vi "Teleop.vi"(10 "Match Info":T1={"Autonomous Elapsed Seconds"=0.0, "TeleOp Elapsed Seconds"=0.0, "Disabled Elapsed Seconds"=0.0, "Visited Autonomous"=FALSE, "Visited TeleOp"=FALSE, "Visited Disabled"=FALSE, "Autonomous Settings"={"Autonomous Style"=enum."Independent", "VI Refnum"=refnum}}, 11 "Call Context":T2) -> ()   [LabVIEW 2013]
doc: "This VI is called for each TeleOp packet received from the DS where the robot is not disabled. It is often used to read from the joysticks and update I/O or to update setpoints for timed control loops. It should complete and return within 20 milliseconds or it may miss DS packets."
uses:
  <vilib>/Rock Robotics/WPI/DriverStation/WPI_DriverStationDerivedRobotMode.ctl
  <vilib>/Rock Robotics/WPI/DriverStation/WPI_DriverStationMatch Info.ctl
  <vilib>/Rock Robotics/WPI/Relay/WPI_RelayValue.ctl
  Robot Global Data.vi
  <vilib>/Rock Robotics/WPI/Joystick/WPI_JoystickGetSetRefNum.vi
  <vilib>/Rock Robotics/WPI/Compressor/WPI_CompressorGetSetRefNum.vi
panel:
  in  "Release to Retract":u32=750
  in  "Time Between Open and Shoot":u32=250
  in  "GO BUTTON?":bool
  out "Numeric 1":dbl(slide) scale=0.0..100.0
  out "Boolean 2":bool
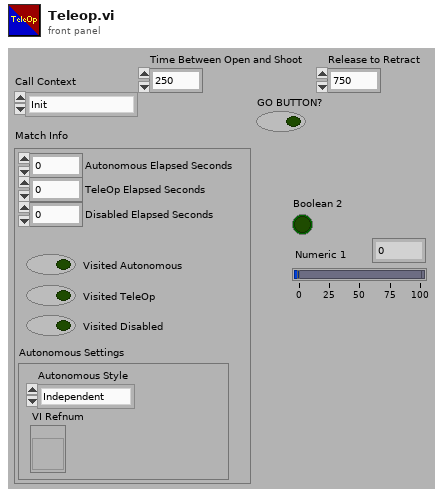
[diagram p1: front panel]
types:
  T1 = typedef "WPI_DriverStationMatch Info.ctl" = cluster{"Autonomous Elapsed Seconds":dbl, "TeleOp Elapsed Seconds":dbl, "Disabled Elapsed Seconds":dbl, "Visited Autonomous":bool, "Visited TeleOp":bool, "Visited Disabled":bool, "Autonomous Settings":cluster{"Autonomous Style":enum16{"Iterative", "Independent"}, "VI Refnum":refnum<vi>}}
  T2 = typedef "WPI_DriverStationDerivedRobotMode.ctl" = enum16{"Init", "Execute", "Stop"}
  T3 = typedef "WPI_RelayValue.ctl" = enum16{"Off", "On", "Forward", "Reverse"}
  T4 = typedef "WPI_JoystickDevRef.ctl" = cluster{"Device":T5}
  T5 = typedef "WPI_JoystickDeviceEnum.ctl" = enum16{"USB 1", "USB 2", "USB 3", "USB 4", "Kinect 1", "Kinect 2"}
  T6 = typedef "WPI_JoystickButtonState.ctl" = cluster{"Button 1":bool, "Button 2":bool, "Button 3":bool, "Button 4":bool, "Button 5":bool, "Button 6":bool, "Button 7":bool, "Button 8":bool, "Button 9":bool, "Button 10":bool, "Button 11":bool, "Button 12":bool}
  T7 = cluster{"axis 1 (x)":dbl, "axis 2 (y)":dbl, "axis 3 (throttle)":dbl, "axis 4":dbl, "axis 5":dbl, "axis 6":dbl}
  T8 = typedef "WPI_RelayDevRef.ctl" = cluster{"DevStatus":errorcluster, "Relay Channel":T9, "Digital Module":T10, "Relay Direction":T11}
  T9 = typedef "FPGA_DIORelayChannel.ctl" = enum8{"Relay 1", "Relay 2", "Relay 3", "Relay 4", "Relay 5", "Relay 6", "Relay 7", "Relay 8", "Invalid"}
  T10 = typedef "FPGA_TypedefDigitalModule.ctl" = enum16{"Digital Module 1", "Digital Module 2"}
  T11 = typedef "WPI_RelayDirection.ctl" = enum16{"Both directions", "Forward only", "Reverse only"}
  T12 = typedef "WPI_CompressorDevRef.ctl" = cluster{"DevStatus":errorcluster, "DigitalInputDevRef":T13, "RelayDevRef":T8}
  T13 = typedef "WPI_DigitalInputDevRef.ctl" = cluster{"DevStatus":errorcluster, "DIO Channel":T14, "Digital Module":T10}
  T14 = typedef "FPGA_DIOChannel.ctl" = enum8{"DIO 1", "DIO 2", "DIO 3", "DIO 4", "DIO 5", "DIO 6", "DIO 7", "DIO 8", "DIO 9", "DIO 10", "DIO 11", "DIO 12", "DIO 13", "DIO 14", "Invalid"}
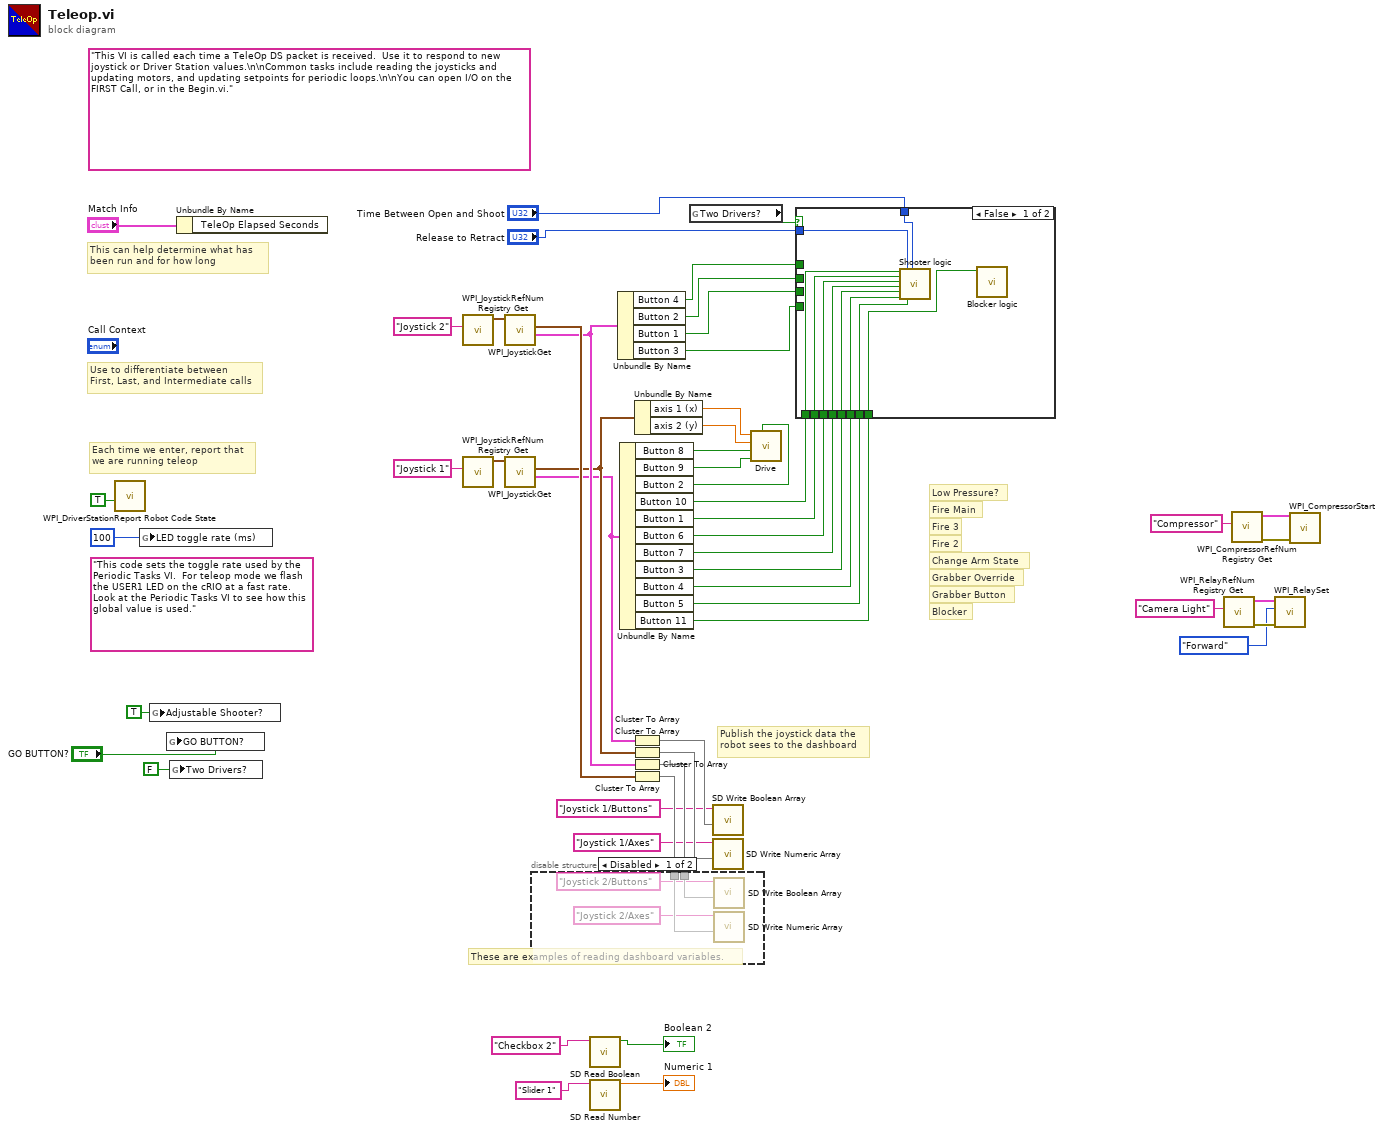
[diagram p0: block diagram]
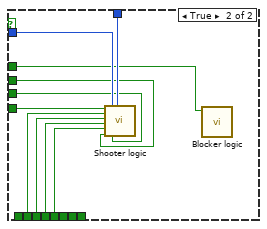
[diagram p2: hidden frame]
diagram:
  (unwired) "This code sets the toggle rate used by the Periodic Tasks VI.  For teleop mode we flash the USER1 LED on the cRIO at a fast rate.  Look at the Periodic Tasks VI to see how this global value is used."
  (unwired) "This VI is called each time a TeleOp DS packet is received.  Use it to respond to new joystick or Driver Station values.\n\nCommon tasks include reading the joysticks and updating motors, and updating setpoints for periodic loops.\n\nYou can open I/O on the FIRST Call, or in the Begin.vi."
  # "Blocker"
  # "Grabber Button"
  # "Grabber Override"
  # "Change Arm State"
  # "Fire 2"
  # "Fire 3"
  # "Fire Main"
  # "Low Pressure?"
  # "These are examples of reading dashboard variables."
  # "Publish the joystick data the\nrobot sees to the dashboard"
  # "Each time we enter, report that\nwe are running teleop"
  # "Use to differentiate between\nFirst, Last, and Intermediate calls"
  # "This can help determine what has\nbeen run and for how long"
  n1 = call <vilib>:"WPI_DriverStationReport Robot Code State.vi"("TeleOp"=TRUE ("Autonomous")) -> ()  [unwired: 10 in, 1 out]
  n2 = global write "Robot Global Data.vi" "LED toggle rate (ms)"(u32 100 ("LED ms toggle rate")) -> ()
  n3 = global write "Robot Global Data.vi" "Adjustable Shooter?"(TRUE ("GO BUTTON?")) -> ()
  n4 = global write "Robot Global Data.vi" "GO BUTTON?"("GO BUTTON?") -> ()
  n5 = global write "Robot Global Data.vi" "Two Drivers?"(FALSE ("GO BUTTON?")) -> ()
  n6 = Unbundle By Name("Match Info") -> ()  [unwired: 1 out]
  n7 = call <vilib>:"WPI_JoystickRefNum Registry Get.vi"("refnum name"="Joystick 2") -> ("JoystickDevRef"=w32:T4)  [unwired: 1 in, 9 out]
  n8 = call <vilib>:"WPI_JoystickRefNum Registry Get.vi"("refnum name"="Joystick 1") -> ("JoystickDevRef"=w49:T4)  [unwired: 1 in, 9 out]
  n9 = call <vilib>:"WPI_JoystickGet.vi"("JoystickDevRef"=w32) -> ("Buttons"=w28:T6, "Axes"=w30:T7)  [unwired: 1 in, 4 out]
  n10 = call <vilib>:"WPI_JoystickGet.vi"("JoystickDevRef"=w49) -> ("Buttons"=w25:T6, "Axes"=w26:T7)  [unwired: 1 in, 4 out]
  n11 = call <vilib>:"SD Read Boolean.vi"("Name"="Checkbox 2" ("refnum name")) -> ("Boolean"=→"Boolean 2":bool)  [unwired: 8 in, 2 out]
  n12 = call <vilib>:"SD Read Number.vi"("Name"="Slider 1" ("refnum name")) -> ("Numeric"=→"Numeric 1":dbl)  [unwired: 8 in, 2 out]
  n13 = Unbundle By Name(w28) -> ("Button 4"=w1:bool, "Button 2"=w5:bool, "Button 1"=w4:bool, "Button 3"=w3:bool)
  n14 = Unbundle By Name(w25) -> ("Button 8"=w38:bool, "Button 9"=w37:bool, "Button 2"=w15:bool, "Button 10"=w12:bool, "Button 1"=w11:bool, "Button 6"=w10:bool, "Button 7"=w9:bool, "Button 3"=w8:bool, "Button 4"=w7:bool, "Button 5"=w6:bool, "Button 11"=w2:bool)
  n15 = Cluster To Array(cluster=w25) -> (array=w46:bool[])
  n16 = Cluster To Array(cluster=w26) -> (array=w45:dbl[])
  n17 = Cluster To Array(cluster=w28) -> (array=w27:bool[])
  n18 = Cluster To Array(cluster=w30) -> (array=w29:dbl[])
  n19 = disable-structure shown="Disabled" {
    disable-tunnel: w29 -> [w55 _]
    disable-tunnel: w27 -> [w54 _]
    frame Disabled {
      n20 = call <vilib>:"SD Write Boolean Array.vi"("Boolean Array"=w54, "Name"="Joystick 2/Buttons") -> ()  [unwired: 8 in, 2 out]
      n21 = call <vilib>:"SD Write Numeric Array.vi"("Numeric Array"=w55, "Name"="Joystick 2/Axes") -> ()  [unwired: 8 in, 2 out]
    }
    frame Enabled {
    }
  }
  n22 = Unbundle By Name(w26) -> ("axis 1 (x)"=w39:dbl, "axis 2 (y)"=w40:dbl)
  n23 = global read "Robot Global Data.vi" "Two Drivers?"() -> (w17:bool)
  n24 = call <vilib>:"SD Write Boolean Array.vi"("Boolean Array"=w46, "Name"="Joystick 1/Buttons") -> ()  [unwired: 8 in, 2 out]
  n25 = call <vilib>:"SD Write Numeric Array.vi"("Numeric Array"=w45, "Name"="Joystick 1/Axes") -> ()  [unwired: 8 in, 2 out]
  n26 = call "Drive.vi"("GO BUTTON"=w15, "Shift up override"=w37, "Shift down override"=w38, "Y axis value"=w40, "X axis value"=w39) -> ()  [unwired: 7 in]
  n27 = case shown="False" w17 {
    tunnel: "Time Between Open and Shoot" -> [w65 w75]
    tunnel: "Release to Retract" -> [w64 w74]
    tunnel: w12 -> [w63 _]
    tunnel: w11 -> [w62 w73]
    tunnel: w10 -> [w61 w72]
    tunnel: w9 -> [w60 w71]
    tunnel: w8 -> [w59 w70]
    tunnel: w7 -> [w58 _]
    tunnel: w6 -> [w57 _]
    tunnel: w4 -> [_ w69]
    tunnel: w5 -> [_ w68]
    tunnel: w3 -> [_ w67]
    tunnel: w2 -> [w56 _]
    tunnel: w1 -> [_ w66]
    frame False {
      n28 = call "Shooter logic.vi"("Low Pressure?"=w63, "Fire Main"=w62, "Fire 3"=w61, "Fire 2"=w60, "Change Arm State"=w59, "Grabber Override"=w58, "Release to Retract"=w64, "Grabber Button"=w57, "Time Between Open and Shoot"=w65) -> ()  [unwired: 11 in]
      n29 = call "Blocker logic.vi"("Botton on"=w56) -> ()  [unwired: 11 in]
    }
    frame True {
      n30 = call "Shooter logic.vi"("Low Pressure?"=w67, "Fire Main"=w73, "Fire 3"=w72, "Fire 2"=w71, "Change Arm State"=w70, "Grabber Override"=w68, "Release to Retract"=w74, "Grabber Button"=w69, "Time Between Open and Shoot"=w75) -> ()  [unwired: 11 in]
      n31 = call "Blocker logic.vi"("Botton on"=w66) -> ()  [unwired: 11 in]
    }
  }
  n32 = call <vilib>:"WPI_RelayRefNum Registry Get.vi"("refnum name"="Camera Light") -> ("error out"=w21:errorcluster, "RelayDevRef"=w20:T8)  [unwired: 9 in]
  n33 = call <vilib>:"WPI_CompressorRefNum Registry Get.vi"("refnum name"="Compressor") -> ("error out"=w36:errorcluster, "CompressorDevRef"=w35:T12)  [unwired: 9 in]
  n34 = call <vilib>:"WPI_RelaySet.vi"("error in (no error)"=w21, "RelayValue"=WPI_RelayValue."Forward", "RelayDevRef"=w20) -> ()  [unwired: 7 in, 2 out]
  n35 = call <vilib>:"WPI_CompressorStart.vi"("error in (no error)"=w36, "CompressorDevRef"=w35) -> ()  [unwired: 8 in, 2 out]
